vi "Autonomous Independent.vi"() -> ()   [LabVIEW 2016]
doc: "This VI is called when autonomous begins, and will automatically be terminated when autonomous ends. You can carry out timed or sensor driven robot movement independently without needing to return to the caller."
uses:
  <vilib>/Rock Robotics/WPI/Utilities/WPI_GetSetVariantRefNum.vi
  <vilib>/Rock Robotics/Network Tables/NT Read String.vi
  <vilib>/Rock Robotics/Network Tables/NT Write Numeric Array.vi
  <vilib>/Rock Robotics/Network Tables/NT Read Boolean.vi
  <vilib>/Rock Robotics/WPI/RobotDrive/WPI_RobotDriveArcadeDrive_Standard(NoSaturation).vi
  Robot Global Data.vi
  AutoaimVar.vi
panel:
  in  "Far Duration":dbl=1.05
  in  "forward Speed 2":dbl=-0.6
  in  "Pivot Speed":dbl=0.5
  in  "Duration":dbl=1.05
  in  "forward Speed":dbl=-0.8
  # "Be sure to right-click and choose Data Operations>>Make Current Value default if you want to save the array values with the VI"
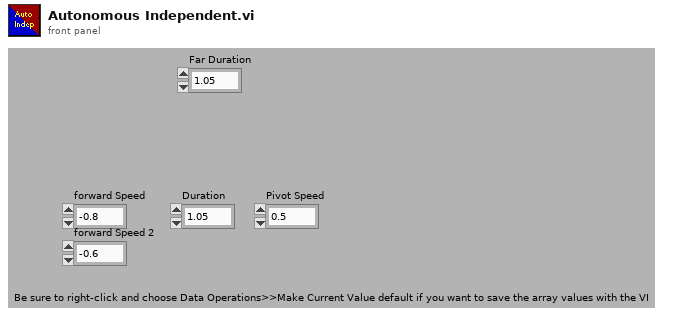
[diagram p1: front panel]
types:
  T1 = typedef "WPI_DriverStationAllianceInfo.ctl" = enum16{"Red", "Blue", "Invalid"}
  T2 = typedef "WPI_DriverStationPositionInfo.ctl" = enum16{"1", "2", "3"}
  T3 = typedef "WPI_JoystickDevRef.ctl" = cluster{"Device":T4}
  T4 = typedef "WPI_JoystickDeviceEnum.ctl" = enum16{"USB 0", "USB 1", "USB 2", "USB 3", "USB 4", "USB 5"}
  T5 = typedef "WPI_RobotDriveDevRef.ctl" = cluster{"DevStatus":errorcluster, "Motors[]":T6[], "Square Inputs":bool, "Max Output":dbl}
  T6 = typedef "WPI_MotorControlDeviceRef.ctl" = cluster{"DeviceStatus":errorcluster, "Type":T7, "PWM":cluster{"PWM Channel":T8, "DeadBand":T9}, "CAN":cluster{"Device Number":u8, "SetOutput VI Ref":variant, "GetOutput VI Ref":variant, "Enable VI Ref":variant, "Disable VI Ref":variant, "Data":variant}, "Invert":bool}
  T7 = typedef "WPI_MotorControlType.ctl" = enum16{"PWM", "CAN"}
  T8 = typedef "FPGA_DIOPWMChannel.ctl" = enum8{"PWM 0", "PWM 1", "PWM 2", "PWM 3", "PWM 4", "PWM 5", "PWM 6", "PWM 7", "PWM 8", "PWM 9", "PWM MXP 0", "PWM MXP 1", "PWM MXP 2", "PWM MXP 3", "PWM MXP 4", "PWM MXP 5", "PWM MXP 6", "PWM MXP 7", "PWM MXP 8", "PWM MXP 9", "Invalid"}
  T9 = typedef "WPI_PWMDeadband.ctl" = cluster{"Name":string, "maxPositivePwm":i32, "minPositivePwm":i32, "centerPwm":i32, "maxNegativePwm":i32, "minNegativePwm":i32, "angularRange":u16}
  T10 = typedef "WPI_GyroDevRef.ctl" = cluster{"DevStatus":errorcluster, "Analog Channel":T11, "Offset":dbl, "Gain (VoltsPerDegree/Second)":dbl, "Gyro Type":enum16{"Analog", "XRS450"}, "Handle":i32, "SPI Bus":T12, "Device Found":bool, "Sample Rate":dbl, "Calibrate On Open":bool}
  T11 = typedef "FPGA_AIChannel.ctl" = enum8{"AI 0", "AI 1", "AI 2", "AI 3", "AI MXP 0", "AI MXP 1", "AI MXP 2", "AI MXP 3", "Invalid"}
  T12 = typedef "spi_bus.ctl" = enum16{"SPI On-Board, CS0", "SPI On-Board, CS1", "SPI On-Board, CS2", "SPI On-Board, CS3", "SPI MXP", "Invalid"}
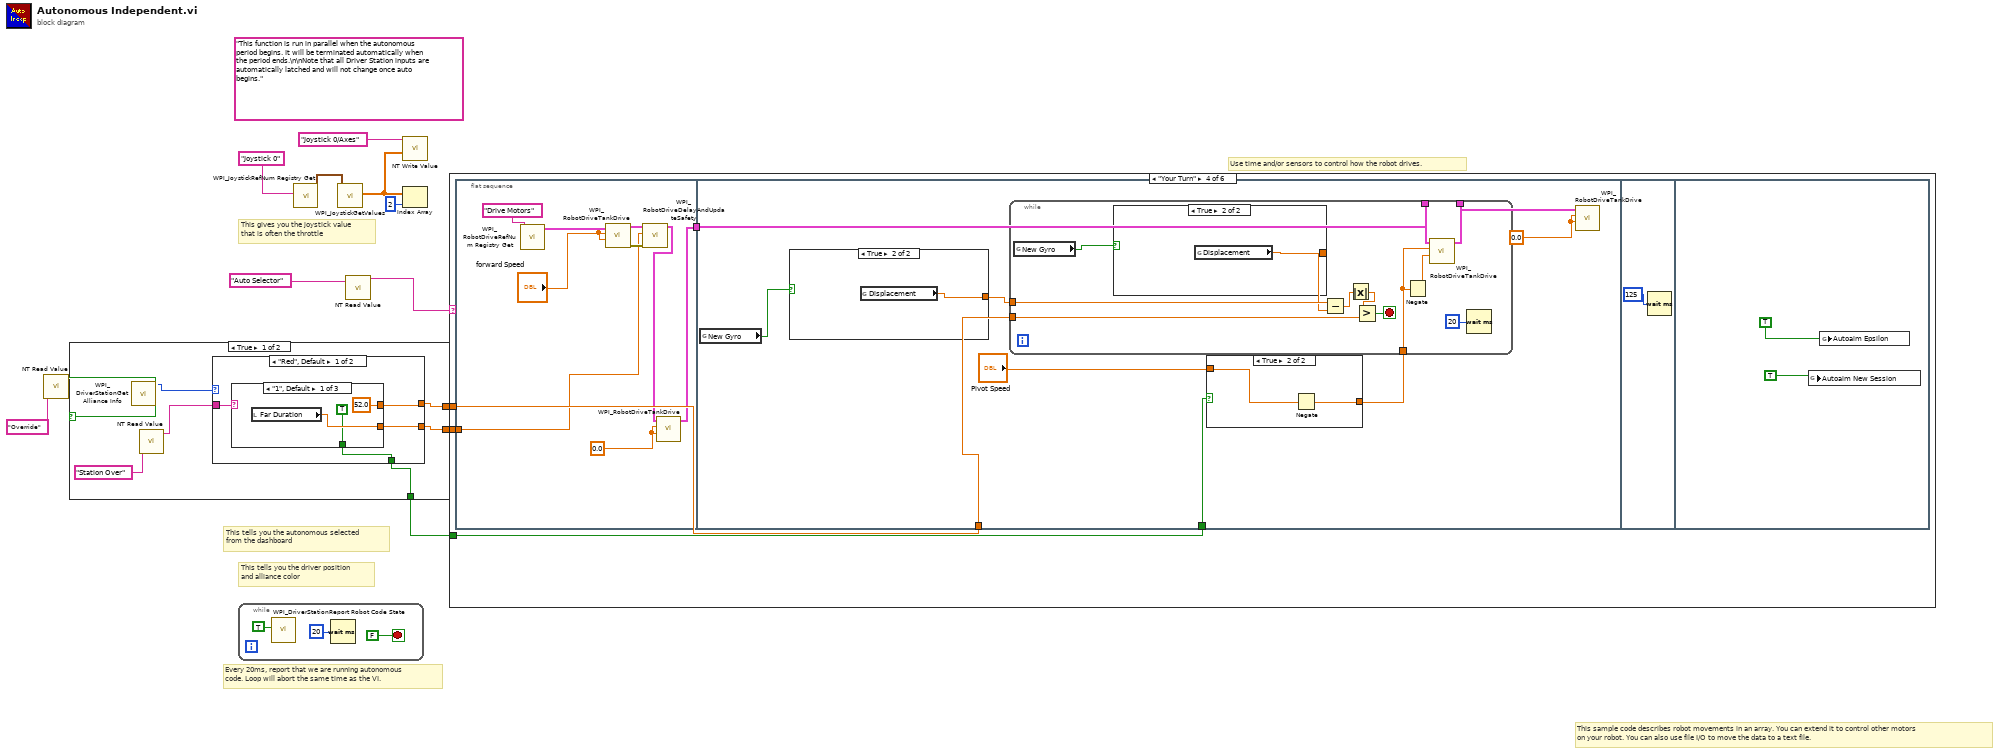
[diagram p0: block diagram]
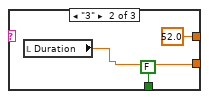
[diagram p2: hidden frame]
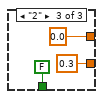
[diagram p3: hidden frame]
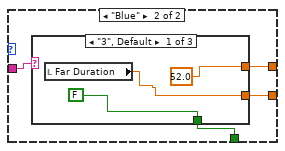
[diagram p4: hidden frame]
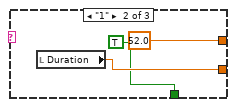
[diagram p5: hidden frame]
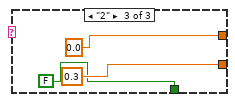
[diagram p6: hidden frame]
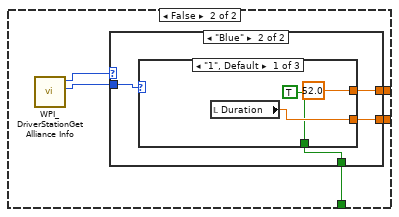
[diagram p7: hidden frame]
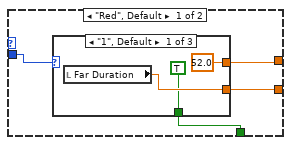
[diagram p8: hidden frame]
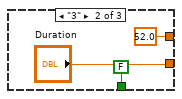
[diagram p9: hidden frame]
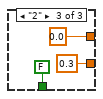
[diagram p10: hidden frame]
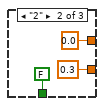
[diagram p11: hidden frame]
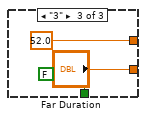
[diagram p12: hidden frame]
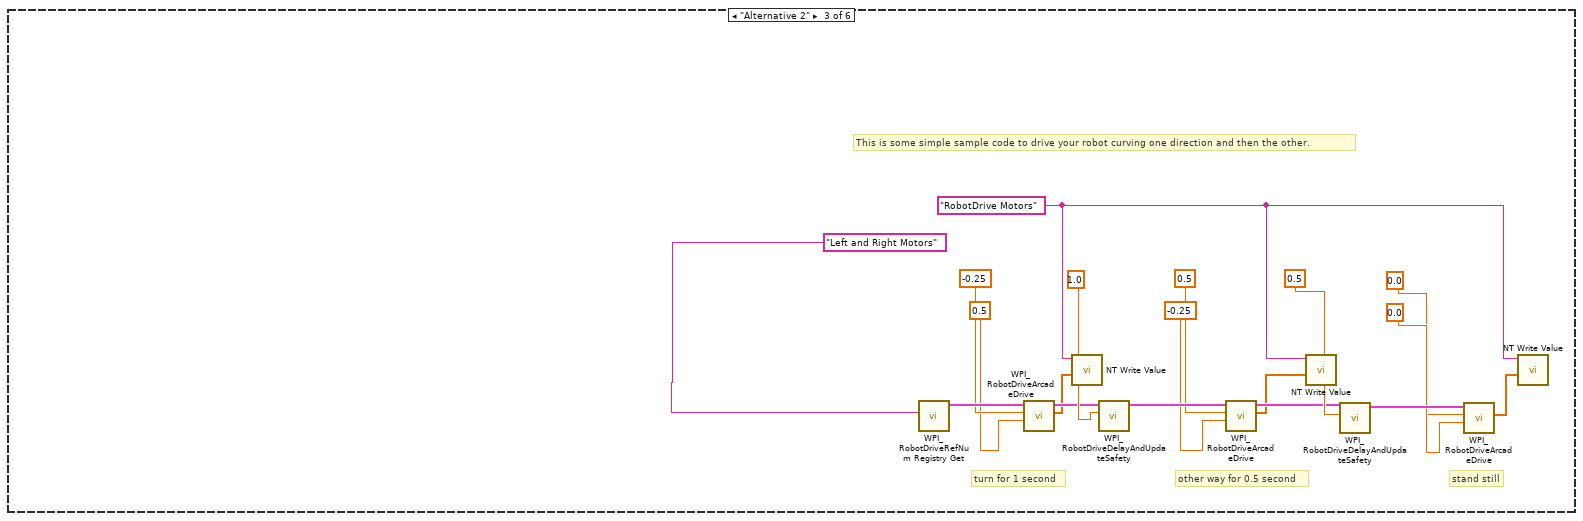
[diagram p15: hidden frame]
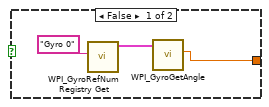
[diagram p16: hidden frame]
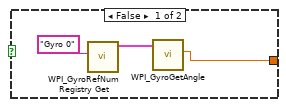
[diagram p17: hidden frame]
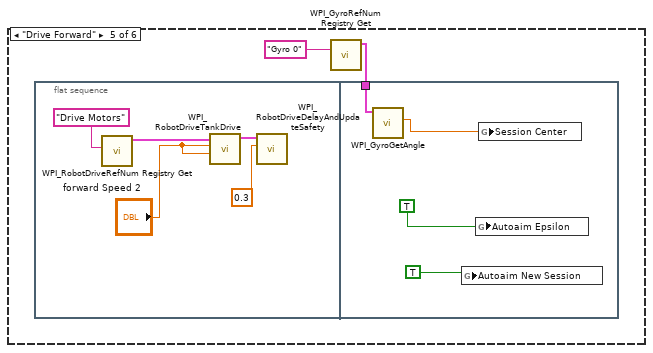
[diagram p19: hidden frame]
diagram:
  (unwired) "This function is run in parallel when the autonomous period begins. It will be terminated automatically when the period ends.\n\nNote that all Driver Station inputs are automatically latched and will not change once auto begins."
  # "This tells you the autonomous selected\nfrom the dashboard"
  # "This sample code describes robot movements in an array. You can extend it to control other motors\non your robot. You can also use file I/O to move the data to a text file."
  # "Every 20ms, report that we are running autonomous\ncode. Loop will abort the same time as the VI."
  # "This gives you the joystick value\nthat is often the throttle"
  # "Use time and/or sensors to control how the robot drives."
  # "This tells you the driver position\nand alliance color"
  n1 = call-poly <vilib>:"NT Read Value.vi"("Name"="Override") -> ("Boolean"=w1:bool)  [unwired: 9 in, 1 out]
  n2 = case shown="True" w1 {
    tunnel: [w17 w47] -> w5
    tunnel: [w18 w46] -> w4
    tunnel: [w13 w45] -> w3
    frame True {
      n3 = call <vilib>:"WPI_DriverStationGet Alliance Info.vi"() -> ("Alliance"=w16:T1)  [unwired: 11 out]
      n4 = call-poly <vilib>:"NT Read Value.vi"("Name"="Station Over") -> ("String"=w14:string)  [unwired: 9 in, 1 out]
      n5 = case shown="\"Red\", Default" w16 {
        tunnel: [w22 w35] -> w17
        tunnel: [w21 w34] -> w18
        tunnel: [w20 w33] -> w13
        tunnel: w14 -> [w19 w32]
        frame "Red", Default {
          n6 = case shown="\"1\", Default" w19 {
            tunnel: [w25 w26 0.3 ("Duration")] -> w22
            tunnel: [52.0 ("y") 52.0 ("y") 0.0 ("y")] -> w21
            tunnel: [TRUE FALSE FALSE] -> w20
            frame "1", Default {
              n7 = local read "Far Duration"() -> (w25:dbl)
            }
            frame "3" {
              n8 = local read "Duration"() -> (w26:dbl)
            }
            frame "2" {
            }
          }
        }
        frame "Blue" {
          n9 = case shown="\"3\", Default" w32 {
            tunnel: [w36 w41 0.3 ("Far Duration")] -> w35
            tunnel: [52.0 ("y") 52.0 ("y") 0.0 ("y")] -> w34
            tunnel: [FALSE TRUE FALSE] -> w33
            frame "3", Default {
              n10 = local read "Far Duration"() -> (w36:dbl)
            }
            frame "1" {
              n11 = local read "Duration"() -> (w41:dbl)
            }
            frame "2" {
            }
          }
        }
      }
    }
    frame False {
      n12 = call <vilib>:"WPI_DriverStationGet Alliance Info.vi"() -> ("Position"=w49:T2, "Alliance"=w48:T1)  [unwired: 10 out]
      n13 = case shown="\"Blue\"" w48 {
        tunnel: w49 -> [w53 w66]
        tunnel: [w52 w65] -> w47
        tunnel: [w51 w64] -> w46
        tunnel: [w50 w63] -> w45
        frame "Red", Default {
          n14 = case shown="\"1\", Default" w53 {
            tunnel: [w56 "Duration" 0.3 ("Duration")] -> w52
            tunnel: [52.0 ("y") 52.0 ("y") 0.0 ("y")] -> w51
            tunnel: [TRUE FALSE FALSE] -> w50
            frame "1", Default {
              n15 = local read "Far Duration"() -> (w56:dbl)
            }
            frame "3" {
            }
            frame "2" {
            }
          }
        }
        frame "Blue" {
          n16 = case shown="\"1\", Default" w66 {
            tunnel: [w69 0.3 ("Far Duration") "Far Duration"] -> w65
            tunnel: [52.0 ("y") 0.0 ("y") 52.0 ("y")] -> w64
            tunnel: [TRUE FALSE FALSE] -> w63
            frame "1", Default {
              n17 = local read "Duration"() -> (w69:dbl)
            }
            frame "2" {
            }
            frame "3" {
            }
          }
        }
      }
    }
  }
  n18 = while {
    stop <- FALSE stop-if-true
    n19 = call <vilib>:"WPI_DriverStationReport Robot Code State.vi"("Autonomous"=TRUE) -> ()  [unwired: 10 in, 1 out]
    n20 = Wait (ms)(milliseconds to wait=u32 20) -> ()  [unwired: 1 out]
  }
  n21 = call <vilib>:"WPI_JoystickRefNum Registry Get.vi"("refnum name"="Joystick 0") -> ("JoystickDevRef"=w11:T3)  [unwired: 1 in, 9 out]
  n22 = call <vilib>:"WPI_JoystickGetValues.vi"("JoystickDevRef"=w11) -> ("Axes"=w7:dbl[])  [unwired: 6 in, 4 out]
  n23 = call-poly <vilib>:"NT Read Value.vi"("Name"="Auto Selector") -> ("String"=w8:string)  [unwired: 9 in, 1 out]
  n24 = call-poly <vilib>:"NT Write Value.vi"("Numeric Array"=w7, "Name"="Joystick 0/Axes") -> ()  [unwired: 9 in, 1 out]
  n25 = Index Array(array=w7, index=2) -> ()  [unwired: 1 out]
  n26 = case shown="\"Your Turn\"" w8 {
    tunnel: w5 -> [_ _ _ w99 _ _]
    tunnel: w4 -> [_ _ _ w98 _ _]
    tunnel: w3 -> [_ _ _ w97 _ _]
    frame Default {
      # "You can put your main auto here, or you can right-click on the case and make any\nother frame be the default case."
      # "This is the frame that will execute if no selection is made, or if it is not recognized"
    }
    frame "Alternative 1" {
    }
    frame "Alternative 2" {
      w79 = "RobotDrive Motors" ("Name")
      # "This is some simple sample code to drive your robot curving one direction and then the other."
      # "stand still"
      # "other way for 0.5 second"
      # "turn for 1 second"
      n27 = call <vilib>:"WPI_RobotDriveRefNum Registry Get.vi"("refnum name"="Left and Right Motors") -> ("RobotDriveDevRef"=w96:T5)  [unwired: 1 in, 9 out]
      n28 = call-poly <vilib>:"WPI_RobotDriveArcadeDrive.vi"("Y axis value"=0.5 ("X axis value"), "X axis value"=-0.25, "RobotDriveDevRef"=w96) -> ("Motor Values"=w80:dbl[], "RobotDriveDevRef"=w89:T5)  [unwired: 1 in, 6 out]
      n29 = call-poly <vilib>:"NT Write Value.vi"("Numeric Array"=w80, "Name"=w79) -> ()  [unwired: 9 in, 1 out]
      n30 = call <vilib>:"WPI_RobotDriveDelayAndUpdateSafety.vi"("Delay (s)"=1.0, "RobotDriveDevRef"=w89) -> ("RobotDriveDevRef 2"=w90:T5)  [unwired: 8 in, 1 out]
      n31 = call-poly <vilib>:"WPI_RobotDriveArcadeDrive.vi"("Y axis value"=-0.25 ("X axis value"), "X axis value"=0.5, "RobotDriveDevRef"=w90) -> ("Motor Values"=w81:dbl[], "RobotDriveDevRef"=w91:T5)  [unwired: 1 in, 6 out]
      n32 = call-poly <vilib>:"NT Write Value.vi"("Numeric Array"=w81, "Name"=w79) -> ()  [unwired: 9 in, 1 out]
      n33 = call <vilib>:"WPI_RobotDriveDelayAndUpdateSafety.vi"("Delay (s)"=0.5, "RobotDriveDevRef"=w91) -> ("RobotDriveDevRef 2"=w92:T5)  [unwired: 8 in, 1 out]
      n34 = call-poly <vilib>:"WPI_RobotDriveArcadeDrive.vi"("Y axis value"=0.0 ("X axis value"), "X axis value"=0.0, "RobotDriveDevRef"=w92) -> ("Motor Values"=w82:dbl[])  [unwired: 1 in, 7 out]
      n35 = call-poly <vilib>:"NT Write Value.vi"("Numeric Array"=w82, "Name"=w79) -> ()  [unwired: 9 in, 1 out]
    }
    frame "Your Turn" {
      n36 = flat-sequence {
        tunnel: [w103] -> w100
        tunnel: w99 -> [w101]
        tunnel: w100 -> [w118]
        tunnel: w98 -> [w112]
        tunnel: w97 -> [w113]
        frame #0 {
          w105 = 0.0 ("Left axis value")
          n37 = call <vilib>:"WPI_RobotDriveRefNum Registry Get.vi"("refnum name"="Drive Motors") -> ("RobotDriveDevRef"=w106:T5)  [unwired: 1 in, 9 out]
          n38 = call <vilib>:"WPI_RobotDriveTankDrive.vi"("Right axis value"="forward Speed", "Left axis value"="forward Speed", "RobotDriveDevRef"=w106) -> ("error out"=w108:errorcluster, "RobotDriveDevRef"=w107:T5)  [unwired: 6 in, 1 out]
          n39 = call <vilib>:"WPI_RobotDriveDelayAndUpdateSafety.vi"("error in (no error)"=w108, "Delay (s)"=w101, "RobotDriveDevRef"=w107) -> ("RobotDriveDevRef 2"=w104:T5)  [unwired: 7 in, 1 out]
          n40 = call <vilib>:"WPI_RobotDriveTankDrive.vi"("Right axis value"=w105, "Left axis value"=w105, "RobotDriveDevRef"=w104) -> ("RobotDriveDevRef"=w103:T5)  [unwired: 6 in, 2 out]
        }
        frame #1 {
          w114 = 0.0 ("Left axis value")
          n41 = global read "Robot Global Data.vi" "New Gyro"() -> (w111:bool)
          n42 = case shown="True" w111 {
            tunnel: [w119 w122] -> w110
            frame False {
              n43 = call <vilib>:"WPI_GyroRefNum Registry Get.vi"("refnum name"="Gyro 0") -> ("GyroDevRef"=w120:T10)  [unwired: 9 in, 1 out]
              n44 = call <vilib>:"WPI_GyroGetAngle.vi"("GyroDevRef"=w120) -> ("Angle"=w119:dbl)  [unwired: 6 in, 4 out]
            }
            frame True {
              n45 = global read "Robot Global Data.vi" "Displacement"() -> (w122:dbl)
            }
          }
          n46 = case shown="True" w113 {
            tunnel: [w139 w141] -> w117
            tunnel: "Pivot Speed" -> [w139 w140]
            frame False {
            }
            frame True {
              n47 = Negate(x=w140) -> (-x=w141:dbl)
            }
          }
          n48 = while {
            tunnel: w110 -> [w134]
            tunnel: w118 -> [w130]
            tunnel: w117 -> [w129]
            tunnel: [w127] -> w115
            tunnel: w112 -> [w125]
            stop <- w133 stop-if-true
            n49 = global read "Robot Global Data.vi" "New Gyro"() -> (w124:bool)
            n50 = case shown="True" w124 {
              tunnel: [w135 w138] -> w123
              frame False {
                n51 = call <vilib>:"WPI_GyroRefNum Registry Get.vi"("refnum name"="Gyro 0") -> ("GyroDevRef"=w136:T10)  [unwired: 9 in, 1 out]
                n52 = call <vilib>:"WPI_GyroGetAngle.vi"("GyroDevRef"=w136) -> ("Angle"=w135:dbl)  [unwired: 6 in, 4 out]
              }
              frame True {
                n53 = global read "Robot Global Data.vi" "Displacement"() -> (w138:dbl)
              }
            }
            n54 = Subtract(x=w134, y=w123) -> (x-y=w132:dbl)
            n55 = Absolute Value(x=w132) -> (abs(x)=w131:dbl)
            n56 = Greater?(x=w131, y=w125) -> (0:w133:bool)
            n57 = Negate(x=w129) -> (-x=w128:dbl)
            n58 = call <vilib>:"WPI_RobotDriveTankDrive.vi"("Right axis value"=w128, "Left axis value"=w129, "RobotDriveDevRef"=w130) -> ("RobotDriveDevRef"=w127:T5)  [unwired: 6 in, 2 out]
            n59 = Wait (ms)(milliseconds to wait=u32 20) -> ()  [unwired: 1 out]
          }
          n60 = call <vilib>:"WPI_RobotDriveTankDrive.vi"("Right axis value"=w114, "Left axis value"=w114, "RobotDriveDevRef"=w115) -> ()  [unwired: 6 in, 3 out]
        }
        frame #2 {
          n61 = Wait (ms)(milliseconds to wait=u32 125) -> ()  [unwired: 1 out]
        }
        frame #3 {
          n62 = global write "AutoaimVar.vi" "Autoaim New Session"(TRUE ("Autoaim New Session")) -> ()
          n63 = global write "AutoaimVar.vi" "Autoaim Epsilon"(TRUE) -> ()
        }
      }
    }
    frame "Drive Forward" {
      n64 = flat-sequence {
        tunnel: w146 -> [w152]
        frame #0 {
          n65 = call <vilib>:"WPI_RobotDriveRefNum Registry Get.vi"("refnum name"="Drive Motors") -> ("RobotDriveDevRef"=w150:T5)  [unwired: 1 in, 9 out]
          n66 = call <vilib>:"WPI_RobotDriveTankDrive.vi"("Right axis value"="forward Speed 2", "Left axis value"="forward Speed 2", "RobotDriveDevRef"=w150) -> ("RobotDriveDevRef"=w149:T5)  [unwired: 6 in, 2 out]
          n67 = call <vilib>:"WPI_RobotDriveDelayAndUpdateSafety.vi"("Delay (s)"=0.3, "RobotDriveDevRef"=w149) -> ()  [unwired: 8 in, 2 out]
        }
        frame #1 {
          n68 = call <vilib>:"WPI_GyroGetAngle.vi"("GyroDevRef"=w152) -> ("Angle"=w154:dbl)  [unwired: 6 in, 4 out]
          n69 = global write "AutoaimVar.vi" "Autoaim New Session"(TRUE ("Autoaim New Session")) -> ()
          n70 = global write "AutoaimVar.vi" "Autoaim Epsilon"(TRUE) -> ()
          n71 = global write "AutoaimVar.vi" "Session Center"(w154) -> ()
        }
      }
      n72 = call <vilib>:"WPI_GyroRefNum Registry Get.vi"("refnum name"="Gyro 0") -> ("GyroDevRef"=w146:T10)  [unwired: 9 in, 1 out]
    }
    frame "Stationary" {
    }
  }
